vi "Get Class A Instances.vi"(8 "error in (no error)":errorcluster, 11 "Lookup in":refnum<data-value>) -> (0 "error out":errorcluster, 3 "Lookup out":refnum<data-value>, 5 "instances of A":refnum<data-value>[](array[refnum]))   [LabVIEW 2014, in "LVCOOOP Tests.lvlib"]
uses:
  LVCOOOP Tests.lvlib
  LVCOOOP/Lookup API/Services/Lookup Service/Lookup Service.lvclass
  Base Class A.lvclass
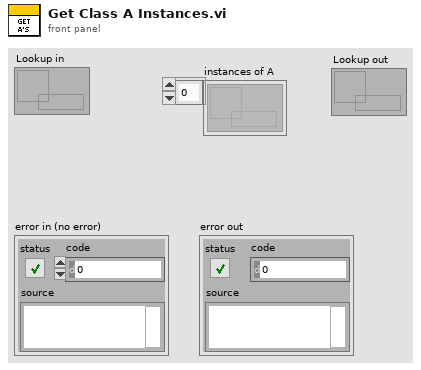
[diagram p1: front panel]
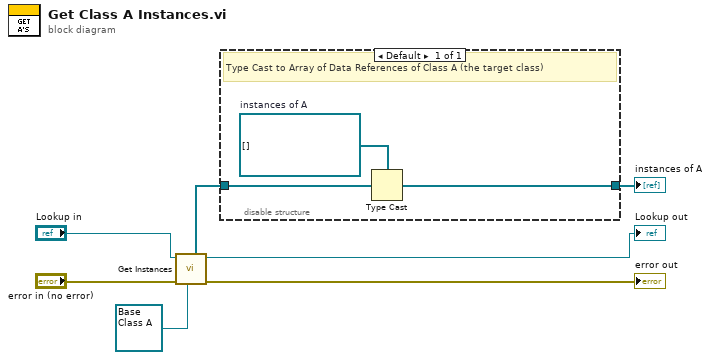
[diagram p0: block diagram]
diagram:
  n1 = call "Get Instances.vi"("Base Class (LabVIEW Object)"=refnum<class "Base Class A.lvclass"> refnum ("LVCOOOP Tests.lvlib:Base Class A.lvclass"), "error in (no error)"="error in (no error)", "Lookup Service in"="Lookup in") -> ("error out"=→"error out":errorcluster, "Lookup Service out"=→"Lookup out":refnum<data-value>, "instances"=w1:refnum<data-value>[])  [unwired: 6 in]
  n2 = disable-structure shown="Default" {
    disable-tunnel: [w9] -> w4
    disable-tunnel: w1 -> [w8]
    frame Enabled {
      w10 = refnum<data-value>[] []  # instances of A
      # "Type Cast to Array of Data References of Class A (the target class)"
      n3 = Type Cast(type=w10, x=w8) -> (*(type *) &x=w9:refnum<data-value>[])
    }
  }
  "instances of A" <- w4
